vi "CMD_09_SetOutV.vi"(9 "Voltage, d":dbl min=0.0 max=4095.0, 11 "VISA resource name":refnum<visa-resource-name>) -> (3 "VISA resource name out":refnum<visa-resource-name>)   [LabVIEW 2017]
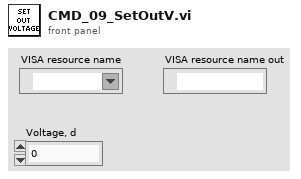
[diagram p1: front panel]
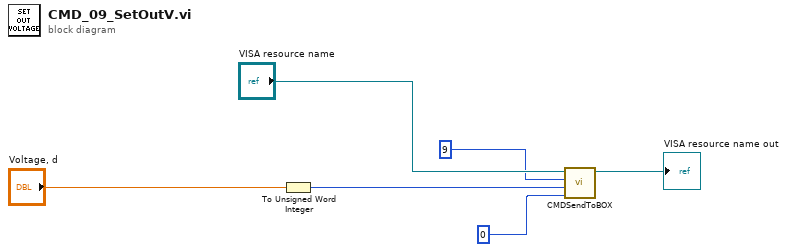
[diagram p0: block diagram]
diagram:
  n1 = To Unsigned Word Integer(number="Voltage, d") -> (unsigned 16bit integer=w3:u16)
  n2 = call "CMDSendToBOX.vi"("arg2"=i16 0, "arg1"=w3, "CMD"=i8 9, "VISA resource name"="VISA resource name") -> ("VISA resource name out"=→"VISA resource name out":refnum<visa-resource-name>)  [unwired: 7 in]
